vi "Digital Output.vi"(0 "VISA resource name":refnum<visa-resource-name>, 5 "Output Channel(s) (121)":string="121", 7 "Digital Value (255)":i32=255, 11 "error in (no error)":errorcluster) -> (4 "VISA resource name out":refnum<visa-resource-name>, 15 "error out":errorcluster)   [LabVIEW 2020, in "Keithley 27XX.lvlib"]
doc: "This VI is used to control the digital output on the selected channels.\n\nNote\n(1) The Model 77xx card being used must support Digital Output to use this VI. \n\n(2) On the 7706 Multiplexer Card there are two 8-bit digital output channels - Ch 21 and Ch 22"
uses:
  Keithley 27XX.lvlib
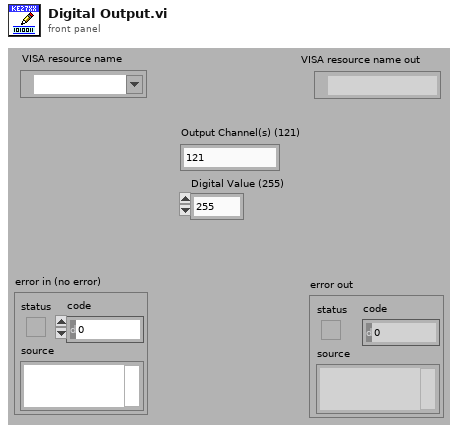
[diagram p1: front panel]
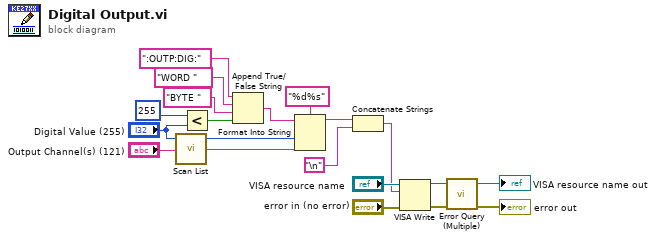
[diagram p0: block diagram]
diagram:
  n1 = call "Scan List.vi"("Scan List (Empty)"="Output Channel(s) (121)") -> ("Scan List Out"=w6:string)  [unwired: 14 in]
  n2 = Less?(x=u32 255 ("y"), y="Digital Value (255)") -> (x < y?=w16:bool)
  n3 = Append True/False String(1:w16, 2:"BYTE " ("false string"), 3:"WORD " ("true string"), 4:":OUTP:DIG:" ("string (\"\")")) -> (0:w7:string)
  n4 = Format Into String(format string="%d%s", initial string=w7, "Digital Value (255)", w6) -> (resulting string=w3:string)  [unwired: 1 in, 1 out]
  n5 = Concatenate Strings(w3, "\n") -> (w2:string)
  n6 = VISA Write(VISA resource name="VISA resource name", write buffer=w2, error in (no error)="error in (no error)") -> (VISA resource name out=w12:refnum<visa-resource-name>, error out=w11:errorcluster)  [unwired: 1 out]
  n7 = call "Error Query (Multiple).vi"("VISA resource name"=w12, "error in (no error)"=w11) -> ("VISA resource name out"=→"VISA resource name out":refnum<visa-resource-name>, "error out"=→"error out":errorcluster)  [unwired: 10 in, 2 out]
